vi "example_01_feedback.vi"() -> ()   [LabVIEW 2015, in "lv-dialog.lvlib"]
uses:
  lv-dialog.lvlib
  _subvis/advanced/feedback-negative.vi
  _subvis/advanced/feedback-positive_negative.vi
  _subvis/advanced/feedback-positive.vi
panel:
  in  "dialog_text_fail":string
  in  "dialog_text_success":string
  out "error out":errorcluster
  in  "error in (no error)":errorcluster
  in  "feedback_selection":T1(radio)
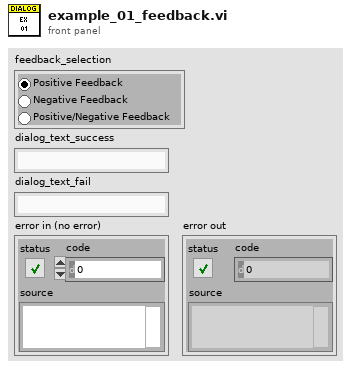
[diagram p1: front panel]
types:
  T1 = enum32{"Positive Feedback", "Negative Feedback", "Positive/Negative Feedback"}
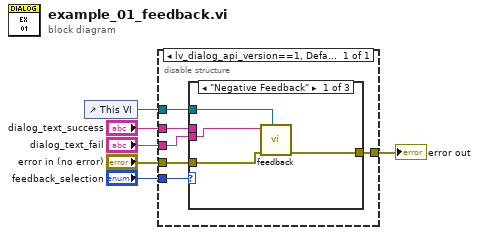
[diagram p0: block diagram]
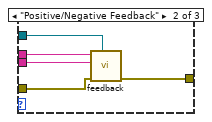
[diagram p2: hidden frame]
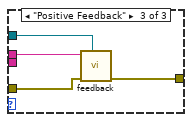
[diagram p3: hidden frame]
diagram:
  n1 = control-ref of="This VI"() -> (w3:refnum<vi>)
  n2 = disable-structure shown="lv_dialog_api_version==1, Default" {
    disable-tunnel: "error in (no error)" -> [w12]
    disable-tunnel: "feedback_selection" -> [w10]
    disable-tunnel: [w11] -> w4
    disable-tunnel: w3 -> [w9]
    disable-tunnel: "dialog_text_success" -> [w8]
    disable-tunnel: "dialog_text_fail" -> [w7]
    frame condition #0 (active) {
      n3 = case shown="\"Negative Feedback\"" w10 {
        tunnel: w12 -> [w13 w17 w22]
        tunnel: [w16 w21 w25] -> w11
        tunnel: w9 -> [w14 w20 w23]
        tunnel: w8 -> [_ w19 w24]
        tunnel: w7 -> [w15 w18 _]
        frame "Negative Feedback" {
          n4 = call-poly "feedback.vi"("callee"=w14, "error in (no error)"=w13, "dialog_text"=w15) -> ("error out"=w16:errorcluster)  [unwired: 8 in]
        }
        frame "Positive/Negative Feedback" {
          n5 = call-poly "feedback.vi"("callee"=w20, "error in (no error)"=w17, "dialog_text_fail"=w18, "dialog_text_success"=w19) -> ("error out"=w21:errorcluster)  [unwired: 7 in]
        }
        frame "Positive Feedback" {
          n6 = call-poly "feedback.vi"("callee"=w23, "error in (no error)"=w22, "dialog_text"=w24) -> ("error out"=w25:errorcluster)  [unwired: 8 in]
        }
      }
    }
  }
  "error out" <- w4
